vi "XY Graph to Igor Graph.vi"(8 "error in (no error)":errorcluster, 9 "Notes":string, 10 "XY Graph Reference":refnum<vi>, 11 "Path":path=path "C:/temp") -> (0 "error out":errorcluster, 3 "file":path=path "C:/Users/voodoo.SEAGATE/Desktop/datatest/datatest.000019.itx")   [LabVIEW 2019, in "Data.ITX.lvclass"]
uses:
  Data.ITX.lvclass
  Graph Utilities/graph_utilities.lvclass
  Data/Data.lvclass
  Data/API/XY-Data to Dictionary (single).vi
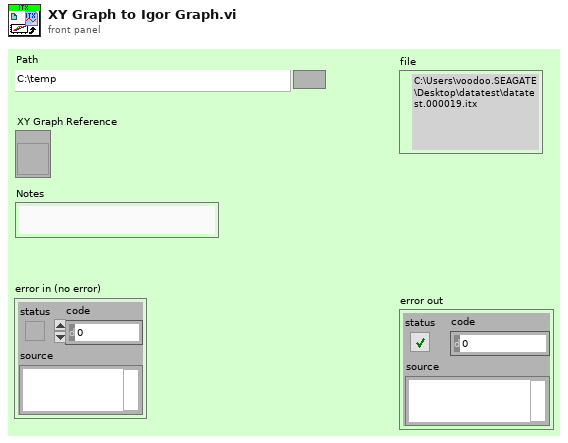
[diagram p1: front panel]
types:
  T1 = typedef "Data.lvclass/Dictionary--cluster.ctl" = cluster{"key":string, "value":variant}
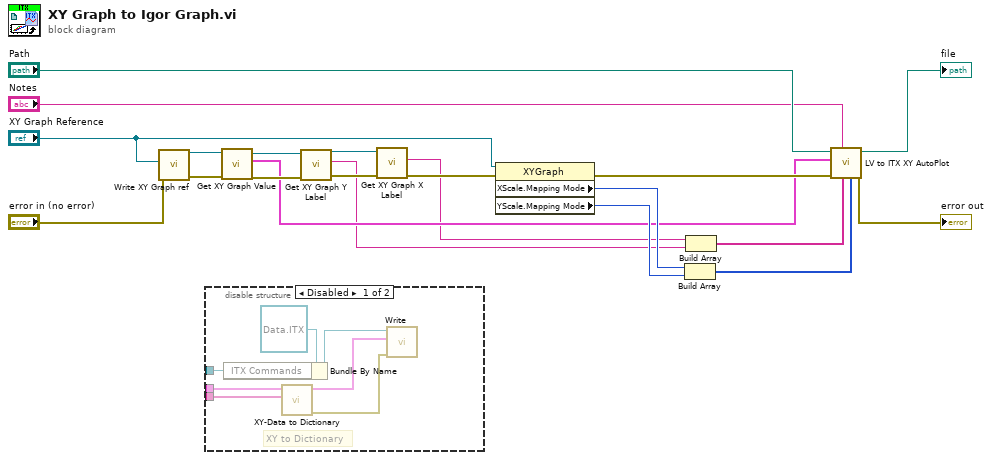
[diagram p0: block diagram]
diagram:
  n1 = call "Write XY Graph ref.vi"("error in (no error)"="error in (no error)", "XY Graph"="XY Graph Reference") -> ("error out"=w20:errorcluster, "graph_utilities out"=w21:refnum<class "graph_utilities.lvclass">)  [unwired: 8 in]
  n2 = disable-structure shown="Disabled" {
    disable-tunnel: _ -> [w26 _]
    disable-tunnel: _ -> [w25 _]
    disable-tunnel: _ -> [w23 _]
    frame Disabled {
      # "XY to Dictionary"
      n3 = Bundle By Name(cluster=refnum<class "Data.ITX.lvclass"> refnum ("Data.ITX in"), "ITX Commands"=w26) -> (w27:refnum<class "Data.ITX.lvclass">)
      n4 = call-poly "XY-Data to Dictionary.vi"("Name"=w23, "XY-data in"=w25) -> ("error out"=w22:errorcluster, "Data (Dictionary)"=w24:T1[])  [unwired: 8 in]
      n5 = call-dynamic "Write.vi"("error in (no error)"=w22, "Data (Dictionary)"=w24, "Data.ITX in"=w27) -> ()  [unwired: 6 in, 3 out]
    }
    frame Enabled {
    }
  }
  n6 = call "Get XY Graph Value.vi"("error in (no error)"=w20, "graph_utilities in"=w21) -> ("error out"=w18:errorcluster, "Value"=w3:cluster{"X":dbl[], "Y":dbl[]}[], "graph_utilities out"=w19:refnum<class "graph_utilities.lvclass">)  [unwired: 7 in]
  n7 = call "Get XY Graph Y Label.vi"("error in (no error)"=w18, "graph_utilities in"=w19) -> ("error out"=w16:errorcluster, "Y Label"=w2:string, "graph_utilities out"=w17:refnum<class "graph_utilities.lvclass">)  [unwired: 7 in]
  n8 = call "Get XY Graph X Label.vi"("error in (no error)"=w16, "graph_utilities in"=w17) -> ("error out"=w15:errorcluster, "X Label"=w1:string)  [unwired: 7 in, 1 out]
  n9 = property on="Property Node" class="XYGraph"(reference="XY Graph Reference", error in=w15) -> (error out=w14:errorcluster, "XScale.Mapping Mode"=w8:u8, "YScale.Mapping Mode"=w7:u8)  [unwired: 1 out]
  n10 = Build Array(w8, w7) -> (w6:u8[])
  n11 = Build Array(w1, w2) -> (w9:string[])
  n12 = call "LV to ITX XY AutoPlot.vi"("X,Y Log"=w6, "X,Y Labels"=w9, "Notes"="Notes", "error in"=w14, "XY-Data []"=w3, "path"="Path") -> ("error out"=→"error out":errorcluster, "file"=→"file":path)  [unwired: 4 in]
